vi "Launch Personalities Tool.vi"() -> (0 "error out":errorcluster)   [LabVIEW 2019, in "Personalities Tool.lvlib"]
uses:
  Main.vi
  Personalities Tool.lvlib
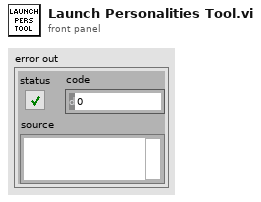
[diagram p1: front panel]
types:
  T1 = enum32{"Invalid", "Standard", "Closed", "Hidden", "Minimized", "Maximized"}
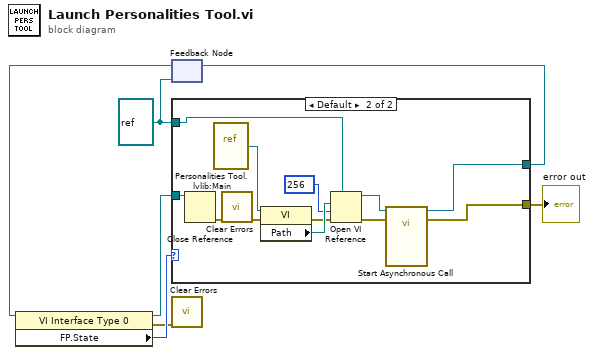
[diagram p0: block diagram]
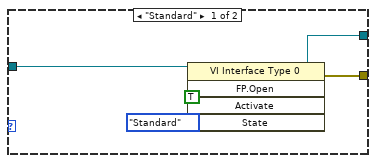
[diagram p2: hidden frame]
diagram:
  w3 = refnum<vi> refnum ("type specifier VI Refnum (for type only)")
  n1 = feedback #1(w3) -> (w4:refnum<vi>)
  n2 = property class="VI Interface Type 0"(reference=w4) -> (reference out=w7:refnum<vi>, error out=w5:errorcluster, "FP.State"=w6:T1)  [unwired: 1 in]
  n3 = case shown="Default" w6 {
    tunnel: [w11 w15] -> w1
    tunnel: [w8 w14] -> w2
    tunnel: w3 -> [_ w23]
    tunnel: w7 -> [w12 w20]
    frame "Standard" {
      n4 = invoke class="VI Interface Type 0" method="FP.Open"(reference=w12, "Activate"=TRUE ("Activate?"), "State"=T1."Standard") -> (reference out=w8:refnum<vi>, error out=w11:errorcluster)  [unwired: 2 in, 3 out]
    }
    frame Default {
      n5 = Close Reference(reference=w20) -> (error out=w21:errorcluster)  [unwired: 1 in]
      n6 = vi-ref "Personalities Tool.lvlib:Main.vi"() -> (w22:refnum<vi>)
      n7 = call <vilib>:"Clear Errors.vi"("error in (no error)"=w21) -> ("error out"=w18:errorcluster)  [unwired: 5 in, 1 out]
      n8 = property class="VI"(reference=w22, error in=w18) -> (error out=w19:errorcluster, "Path"=w24:path)  [unwired: 1 out]
      n9 = Open VI Reference(type specifier VI Refnum (for type only)=w23, vi path=w24, options=256, error in (no error)=w19) -> (vi reference=w16:refnum<vi>, error out=w17:errorcluster)  [unwired: 2 in]
      n10 = call-by-ref "Start Asynchronous Call"(reference=w16, error in=w17) -> (reference out=w14:refnum<vi>, error out=w15:errorcluster)  [unwired: 12 in]
    }
  }
  "error out" <- w1
  n11 = feedback-in #1(w2) -> ()
  n12 = call <vilib>:"Clear Errors.vi"("error in (no error)"=w5) -> ()  [unwired: 5 in, 2 out]
